vi "User Event Init.vi"() -> (2 "Event Registration Refnum":refnum<event-registration>, 3 "user events":T1)   [LabVIEW 2021, in "TSC Button Editor.lvclass"]
doc: "create user events for the button editor.\n\n<b>Code Developed By:</b> +\nDaniel Coons +\nTechnology Service Corporation +\nwww.tsc.com/atcs"
uses:
  TSC Button Editor.lvclass
  User Events--typedef.ctl
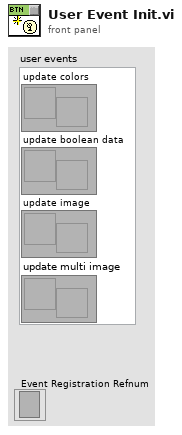
[diagram p1: front panel]
types:
  T1 = typedef "TSC Button Editor.lvclass/User Events--typedef.ctl" = cluster{"update colors":refnum<user-event>, "update boolean data":refnum<user-event>, "update image":refnum<user-event>, "update multi image":refnum<user-event>}
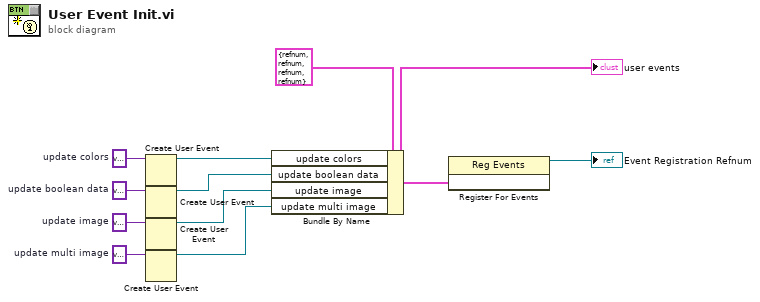
[diagram p0: block diagram]
diagram:
  w2 = variant  # update multi image
  w4 = variant  # update image
  w11 = variant  # update boolean data
  w10 = variant  # update colors
  n1 = Create User Event(user event datatype=w10) -> (user event=w7:refnum<user-event>)  [unwired: 1 in, 1 out]
  n2 = Create User Event(user event datatype=w11) -> (user event=w8:refnum<user-event>)  [unwired: 1 in, 1 out]
  n3 = Create User Event(user event datatype=w4) -> (user event=w3:refnum<user-event>)  [unwired: 1 in, 1 out]
  n4 = Create User Event(user event datatype=w2) -> (user event=w1:refnum<user-event>)  [unwired: 1 in, 1 out]
  n5 = Bundle By Name(cluster=T1 {"update colors"=refnum, "update boolean data"=refnum, "update image"=refnum, "update multi image"=refnum}, "update colors"=w7, "update boolean data"=w8, "update image"=w3, "update multi image"=w1) -> (w6:T1)
  "user events" <- w6
  n6 = register-events(w6) -> (reference out=→"Event Registration Refnum":refnum<event-registration>)  [unwired: 2 in, 1 out]
